vi "Air Constants.vi"() -> ()   [LabVIEW 2020]
uses:
  Air Flow State.ctl
  School Work/Internship I/LabVIEW Data/Gas Turbine Condition Plotter/Utilities/Time Stamp.ctl
  Combined State.ctl
panel:
  in  "Tab Control":enum32{"Constants", "Default Unknown State"}(tab)=enum."Default Unknown State"
  in  "Default Combined State":T1={"Default Unknown Air State"={"Flow Rate [CFM]"=0.0, "Pressure [psia]"=0.0, "Dry Bulb Temp [DegF]"=-460.0, "Wet Bulb Temp [DegF]"=-460.0, "Relative Humidity [%]"=-460.0, "Humidity Ratio [lbmv/lbma]"=-460.0, "Grains [Gr/lbma]"=-460.0, "Specific Volume [ft^3/lbma]"=-460.0, "Enthalpy [BTU/lbm]"=-460.0, "Dew Point [DegF]"=-460.0}, "Default Unknown Time Stamp"={"Year"=0, "Month"=0, "Day"=0, "Hour"=0, "Minute"=0}}
  in  "Default Unknown Time Stamp":T3
  in  "Default Unknown Air State":T2={"Flow Rate [CFM]"=0.0, "Pressure [psia]"=0.0, "Dry Bulb Temp [DegF]"=-460.0, "Wet Bulb Temp [DegF]"=-460.0, "Relative Humidity [%]"=-460.0, "Humidity Ratio [lbmv/lbma]"=-460.0, "Grains [Gr/lbma]"=-460.0, "Specific Volume [ft^3/lbma]"=-460.0, "Enthalpy [BTU/lbm]"=-460.0, "Dew Point [DegF]"=-460.0}
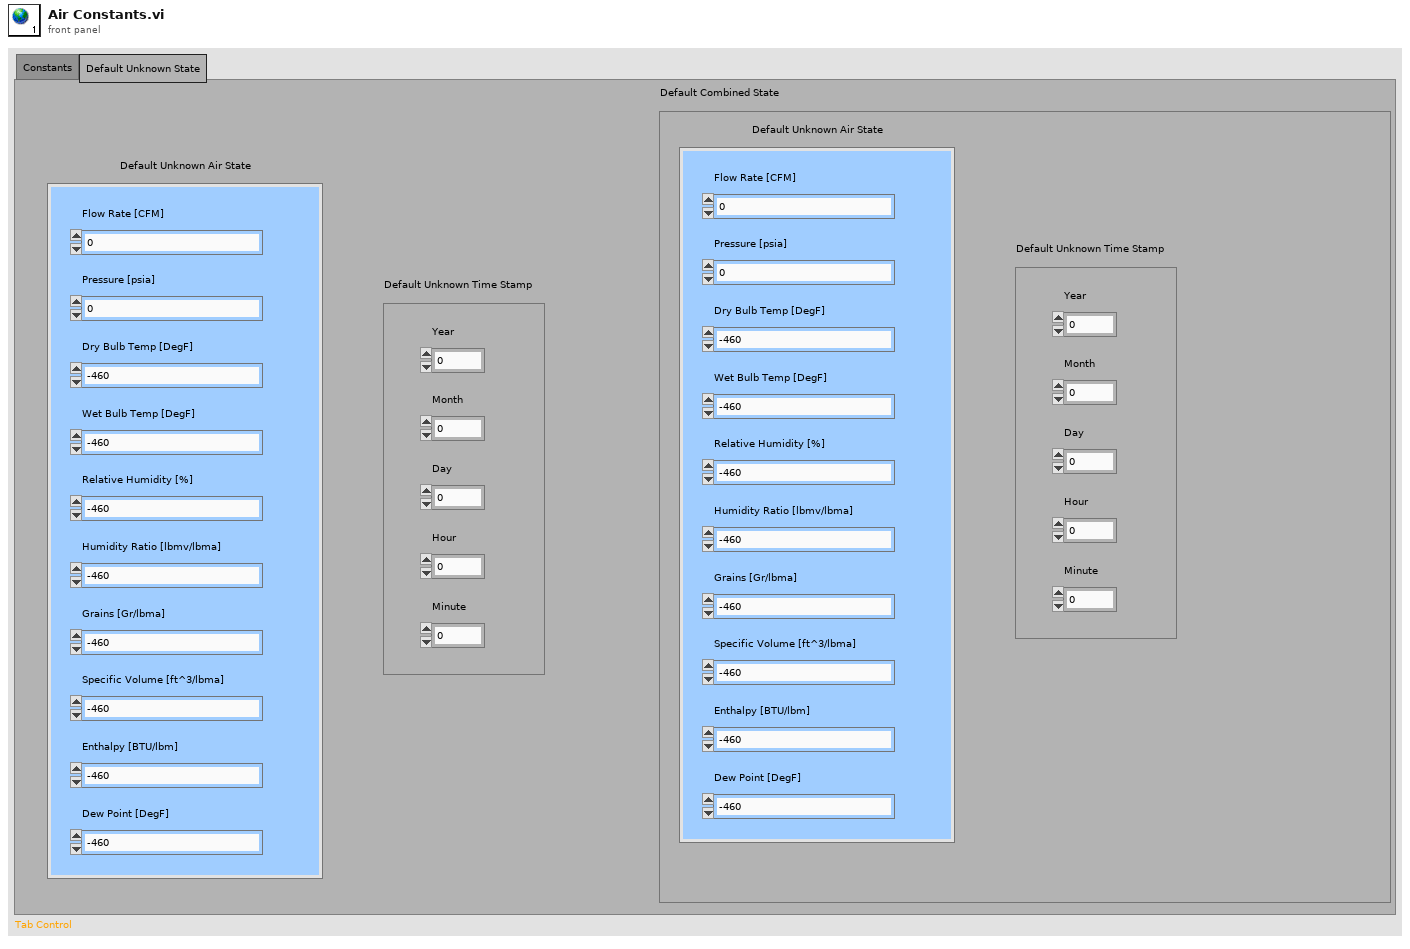
[diagram p1: front panel]
types:
  T1 = typedef "Combined State.ctl" = cluster{"Default Unknown Air State":T2, "Default Unknown Time Stamp":T3}
  T2 = typedef "Air Flow State.ctl" = cluster{"Flow Rate [CFM]":dbl, "Pressure [psia]":dbl, "Dry Bulb Temp [DegF]":dbl, "Wet Bulb Temp [DegF]":dbl, "Relative Humidity [%]":dbl, "Humidity Ratio [lbmv/lbma]":dbl, "Grains [Gr/lbma]":dbl, "Specific Volume [ft^3/lbma]":dbl, "Enthalpy [BTU/lbm]":dbl, "Dew Point [DegF]":dbl}
  T3 = typedef "Time Stamp.ctl" = cluster{"Year":i32, "Month":i32, "Day":i32, "Hour":i32, "Minute":i32}
diagram:
